vi "WaitForShooter.vi"(8 "error in (no error)":errorcluster, 11 "State":T1) -> (0 "error out":errorcluster, 3 "Timeout":bool)   [LabVIEW 2013]
uses:
  ShooterStates.ctl
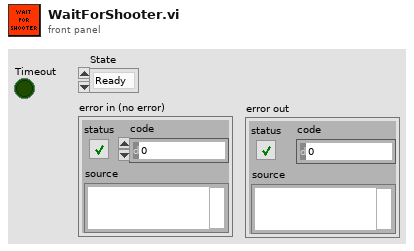
[diagram p1: front panel]
types:
  T1 = typedef "ShooterStates.ctl" = enum16{"Ready", "RetractFull", "Disengage Clutch", "Clutch Delay", "Fire", "Fire Delay", "Latch", "Retract", "Release", "Setup"}
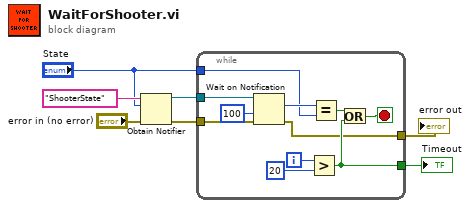
[diagram p0: block diagram]
diagram:
  n1 = Obtain Notifier(name (unnamed)="ShooterState", notification data type="State", error in (no error)="error in (no error)") -> (notifier out=w5:refnum<notifier>, error out=w3:errorcluster)  [unwired: 1 in, 1 out]
  n2 = while {
    tunnel: [w12] -> w7
    tunnel: w5 -> [w11]
    tunnel: "State" -> [w10]
    tunnel: w3 -> [w9]
    tunnel: [w8] -> w1
    i -> [w14]
    stop <- w15 stop-if-true
    n3 = Wait on Notification(notifier=w11, timeout in ms (-1)=100, error in (no error)=w9) -> (notification=w17:T1, error out=w8:errorcluster)  [unwired: 1 in, 2 out]
    n4 = Greater?(x=w14, y=20) -> (0:w12:bool)
    n5 = Equal?(x=w17, y=w10) -> (x = y?=w16:bool)
    n6 = Or(x=w16, y=w12) -> (x .or. y?=w15:bool)
  }
  "Timeout" <- w7
  "error out" <- w1
